vi "Write CAN Frame.vi"(7 "CAN Channel":u16=1, 8 "error in (no error)":errorcluster, 10 "CAN Frame":T1 {"type" items=["CAN Data"=0, "CAN Remote"=1, "CAN Bus Error"=2, "CAN 2.0 Data"=8, "CAN FD Data"=16, "CAN FD+BRS Data"=24, "J1939 Data"=192, "Delay"=224, "Log Trigger"=225, "Start Trigger"=226]; "payload" format="%x"; "timestamp" format="%<%.7X\n%x>T"; "identifier" format="%x"}, 11 "BLF File In":refnum<class "Read Write BLF.lvclass">) -> (0 "error out":errorcluster, 3 "BLF File Out":refnum<class "Read Write BLF.lvclass">)   [LabVIEW 2015, in "Read Write BLF.lvclass"]
doc: "This VI will write a single <B>CAN frame</B> to a BLF File.\n\n-------------\nBrian Hoover (Hooovahh)"
uses:
  Read Write BLF.lvclass
  Controls/Cluster - CAN Frame.ctl
  Controls/Enum - CAN Data Type.ctl
  Read Write BLF.lvclass/Read Write BLF.ctl
  Controls/Cluster - CAN Message.ctl
  Controls/Cluster - mHeader.ctl
  Controls/Cluster - mHeaderBase.ctl
  Controls/Enum - Read Object Types.ctl
  <vilib>/Utility/error.llb/Error Cluster From Error Code.vi
  <vilib>/Utility/libraryn.llb/Check if File or Folder Exists.vi
  SubVIs/BasicAppPath.vi
  <vilib>/ErrorRing/Error Ring.xnode
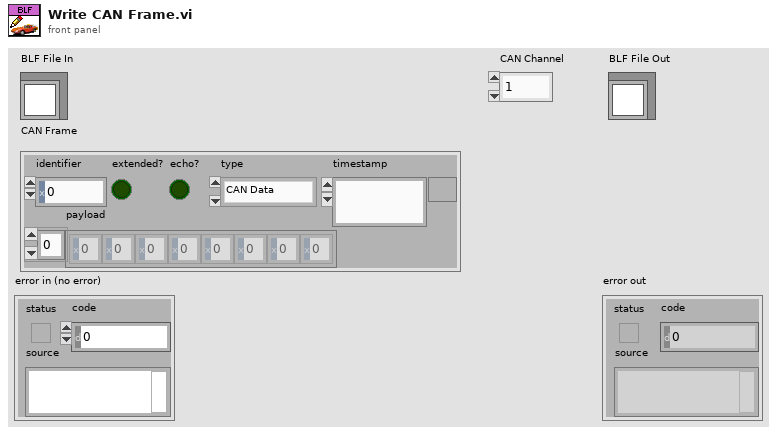
[diagram p1: front panel]
types:
  T1 = typedef "Read Write BLF.lvclass/Cluster - CAN Frame.ctl" = cluster{"timestamp":timestamp, "payload":u8[], "identifier":u32, "extended?":bool, "echo?":bool, "type":T2}
  T2 = typedef "Read Write BLF.lvclass/Enum - CAN Data Type.ctl" = u8
  T3 = typedef "Read Write BLF.lvclass/Cluster - mHeader.ctl" = cluster{"mHeaderBase":T4, "mObjectFlags":u32, "mReserved":u16, "mObjectVersion":u16, "mObjectTimeStamp":u64}
  T4 = typedef "Read Write BLF.lvclass/Cluster - mHeaderBase.ctl" = cluster{"mSignature":u32, "mHeaderSize":u16, "mHeaderVersion":u16, "mObjectSize":u32, "Object Type":T5}
  T5 = typedef "Read Write BLF.lvclass/Enum - Read Object Types.ctl" = enum32{"UNKNOWN", "CAN_MESSAGE", "CAN_ERROR", "CAN_OVERLOAD", "CAN_STATISTIC", "APP_TRIGGER", "ENV_INTEGER", "ENV_DOUBLE", "ENV_STRING", "ENV_DATA", "LOG_CONTAINER", "LIN_MESSAGE", "LIN_CRC_ERROR", "LIN_DLC_INFO", "LIN_RCV_ERROR", "LIN_SND_ERROR", "LIN_SLV_TIMEOUT", "LIN_SCHED_MODCH", "LIN_SYN_ERROR", "LIN_BAUDRATE", "LIN_SLEEP", "LIN_WAKEUP", "MOST_SPY", "MOST_CTRL", "MOST_LIGHTLOCK", "MOST_STATISTIC", "reserved_1", "reserved_2", "reserved_3", "FLEXRAY_DATA", "FLEXRAY_SYNC", "CAN_DRIVER_ERROR", "MOST_PKT", "MOST_PKT2", "MOST_HWMODE", "MOST_REG", "MOST_GENREG", "MOST_NETSTATE", "MOST_DATALOST", "MOST_TRIGGER", "FLEXRAY_CYCLE", "FLEXRAY_MESSAGE", "LIN_CHECKSUM_INFO", "LIN_SPIKE_EVENT", "CAN_DRIVER_SYNC", "FLEXRAY_STATUS", "GPS_EVENT", "FR_ERROR", "FR_STATUS", "FR_STARTCYCLE", "FR_RCVMESSAGE", "REALTIMECLOCK", "AVAILABLE2", "AVAILABLE3", "LIN_STATISTIC", "J1708_MESSAGE", "J1708_VIRTUAL_MSG", "LIN_MESSAGE2", "LIN_SND_ERROR2", "LIN_SYN_ERROR2", "LIN_CRC_ERROR2", "LIN_RCV_ERROR2", "LIN_WAKEUP2", "LIN_SPIKE_EVENT2", "LIN_LONG_DOM_SIG", "APP_TEXT", "FR_RCVMESSAGE_EX", "MOST_STATISTICEX", "MOST_TXLIGHT", "MOST_ALLOCTAB", "MOST_STRESS", "ETHERNET_FRAME", "SYS_VARIABLE", "CAN_ERROR_EXT", "CAN_DRIVER_ERROR_EXT", "LIN_LONG_DOM_SIG2", "MOST_150_MESSAGE", "MOST_150_PKT", "MOST_ETHERNET_PKT", "MOST_150_MESSAGE_FRAGMENT", "MOST_150_PKT_FRAGMENT", "MOST_ETHERNET_PKT_FRAGMENT", "MOST_SYSTEM_EVENT", "MOST_150_ALLOCTAB", "MOST_50_MESSAGE", "MOST_50_PKT", "CAN_MESSAGE2", "LIN_UNEXPECTED_WAKEUP", "LIN_SHORT_OR_SLOW_RESPONSE", "LIN_DISTURBANCE_EVENT", "SERIAL_EVENT", "OVERRUN_ERROR", "EVENT_COMMENT", "WLAN_FRAME", "WLAN_STATISTIC", "MOST_ECL", "GLOBAL_MARKER", "AFDX_FRAME", "AFDX_STATISTIC", "KLINE_STATUSEVENT", "CAN_FD_MESSAGE", "CAN_FD_MESSAGE_64", "ETHERNET_RX_ERROR", "ETHERNET_STATUS", "CAN_FD_ERROR_64", "LIN_SHORT_OR_SLOW_RESPONSE2", "AFDX_STATUS", "AFDX_BUS_STATISTIC"}
  T6 = typedef "Read Write BLF.lvclass/Cluster - CAN Message.ctl" = cluster{"mHeader":T3, "mChannel":u16, "mFlags":u8, "mDLC":u8, "mID":u32, "mData":cluster{"mData[0]":u8, "mData[1]":u8, "mData[2]":u8, "mData[3]":u8, "mData[4]":u8, "mData[5]":u8, "mData[6]":u8, "mData[7]":u8}}
  T7 = cluster{"payload[0]":u8, "payload[1]":u8, "payload[2]":u8, "payload[3]":u8, "payload[4]":u8, "payload[5]":u8, "payload[6]":u8, "payload[7]":u8}
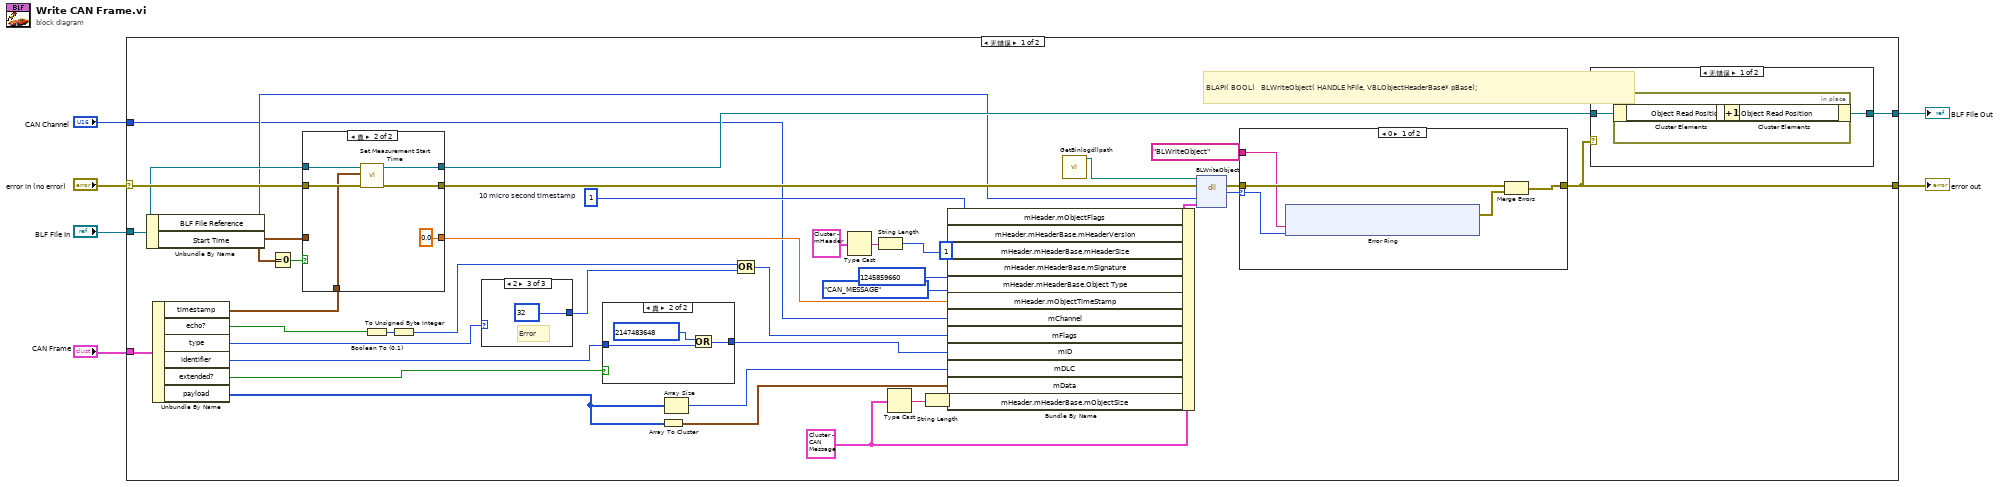
[diagram p0: block diagram]
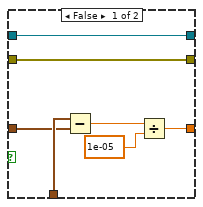
[diagram p2: hidden frame]
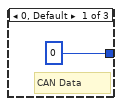
[diagram p3: hidden frame]
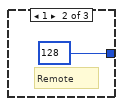
[diagram p4: hidden frame]
diagram:
  n1 = case shown="无错误" "error in (no error)" {
    selector: "error in (no error)" -> [w46 w87]
    tunnel: [w30 w87] -> w5
    tunnel: "CAN Frame" -> [w41 _]
    tunnel: "BLF File In" -> [w12 w86]
    tunnel: [w31 w86] -> w2
    tunnel: "CAN Channel" -> [w8 _]
    frame No Error {
      w15 = u8 1  # 10 micro second timestamp
      w16 = T6 {"mHeader"={"mHeaderBase"={"mSignature"=0, "mHeaderSize"=0, "mHeaderVersion"=0, "mObjectSize"=0, "Object Type"=enum."UNKNOWN"}, "mObjectFlags"=0, "mReserved"=0, "mObjectVersion"=0, "mObjectTimeStamp"=0}, "mChannel"=0, "mFlags"=0, "mDLC"=8, "mID"=0, "mData"={"mData[0]"=0, "mData[1]"=0, "mData[2]"=0, "mData[3]"=0, "mData[4]"=0, "mData[5]"=0, "mData[6]"=0, "mData[7]"=0}}
      # "BLAPI( BOOL)   BLWriteObject( HANDLE hFile, VBLObjectHeaderBase* pBase);"
      n2 = Unbundle By Name(w12) -> ("BLF File Reference"=w9:u32, "Start Time"=w14:timestamp)
      n3 = Unbundle By Name(w41) -> ("timestamp"=w34:timestamp, "echo?"=w29:bool, "type"=w27:T2, "identifier"=w40:u32, "extended?"=w39:bool, "payload"=w36:u8[])
      n4 = Equal To 0?(x=w14) -> (x = 0?=w10:bool)
      n5 = case shown="真" w10 {
        tunnel: w46 -> [w53 w58]
        tunnel: w34 -> [w52 w54]
        tunnel: [w49 0.0] -> w33
        tunnel: w14 -> [w48 _]
        tunnel: [w53 w56] -> w13
        tunnel: w12 -> [w47 w59]
        tunnel: [w47 w57] -> w11
        frame False {
          n6 = Subtract(x=w52, y=w48) -> (x-y=w51:dbl)
          n7 = Divide(x=w51, y=1e-05) -> (x/y=w49:dbl)
        }
        frame True {
          n8 = call "Set Measurement Start Time.vi"("error in (no error)"=w58, "Time Stamp (now)"=w54, "BLF File In"=w59) -> ("error out"=w56:errorcluster, "BLF File Out"=w57:refnum<class "Read Write BLF.lvclass">)  [unwired: 7 in]
        }
      }
      n9 = Boolean To (0,1)(Boolean=w29) -> (0, 1=w28:i16)
      n10 = To Unsigned Byte Integer(number=w28) -> (unsigned 8bit integer=w26:u8)
      n11 = case shown="2" w27 {
        tunnel: [u8 0 u8 128 u8 32] -> w25
        frame 0, Default {
          # "CAN Data"
        }
        frame 1 {
          # "Remote"
        }
        frame 2 {
          # "Error"
        }
      }
      n12 = case shown="真" w39 {
        tunnel: w40 -> [w68 w71]
        tunnel: [w68 w70] -> w38
        frame False {
        }
        frame True {
          n13 = Or(x=u32 2147483648, y=w71) -> (x .or. y?=w70:u32)
        }
      }
      n14 = Array To Cluster(array=w36) -> (cluster=w35:T7)
      n15 = Array Size(array=w36) -> (size(s)=w37:i32)
      n16 = Compound Arithmetic op=OR(w26, w25) -> (w32:u8)
      n17 = Type Cast(x=T3 {"mHeaderBase"={"mSignature"=0, "mHeaderSize"=0, "mHeaderVersion"=0, "mObjectSize"=0, "Object Type"=enum."UNKNOWN"}, "mObjectFlags"=0, "mReserved"=0, "mObjectVersion"=0, "mObjectTimeStamp"=0} ("mHeader")) -> (*(type *) &x=w22:string)  [unwired: 1 in]
      n18 = String Length(string=w22) -> (length=w21:i32)
      n19 = Type Cast(x=w16) -> (*(type *) &x=w18:string)  [unwired: 1 in]
      n20 = String Length(string=w18) -> (length=w17:i32)
      n21 = Bundle By Name(cluster=w16, "mHeader.mObjectFlags"=w15, "mHeader.mHeaderBase.mHeaderVersion"=u16 1, "mHeader.mHeaderBase.mHeaderSize"=w21, "mHeader.mHeaderBase.mSignature"=u32 1245859660, "mHeader.mHeaderBase.Object Type"=Enum_-_Read_Object_Types."CAN_MESSAGE", "mHeader.mObjectTimeStamp"=w33, "mChannel"=w8, "mFlags"=w32, "mID"=w38, "mDLC"=w37, "mData"=w35, "mHeader.mHeaderBase.mObjectSize"=w17) -> (w42:T6)
      n22 = call "GetBinlogdllpath.vi"() -> ("dup path"=w7:path)  [unwired: 11 in]
      n23 = dll-call lib="PTH2Vabs E自开发软件X-CAN项目 X-CAN离线分析平台 V2.2.8.0BLFbinlog.*" fn="BLWriteObject"(path in=w7, error in=w13, "hFile"=w9, "pBase"=w42) -> (error out=w44:errorcluster, "return type"=w43:i32)  [unwired: 3 in, 1 out]
      n24 = case shown="0" w43 {
        selector: w43 -> [w74 _]
        tunnel: w44 -> [w76 w85]
        tunnel: [w75 w85] -> w30
        tunnel: "BLWriteObject" -> [w73 _]
        frame 0 {
          n25 = xnode "Error Ring"("参数 0"=w73, "参数 1"=w74) -> ("错误输出"=w72:errorcluster)
          n26 = Merge Errors(w76, w72) -> (w75:errorcluster)
        }
        frame Default {
        }
      }
      n27 = case shown="无错误" w30 {
        tunnel: w11 -> [w64 w67]
        tunnel: [w63 w67] -> w31
        frame No Error {
          n28 = in-place {
            n29 = in-place-cluster #1(w64) -> ("Object Read Position"=w66:u32)
            n30 = Increment(x=w66) -> (x+1=w65:u32)
            n31 = in-place-cluster #1("Object Read Position"=w65) -> (w63:refnum<class "Read Write BLF.lvclass">)
          }
        }
        frame Error {
        }
      }
    }
    frame Error {
    }
  }
  "error out" <- w5
  "BLF File Out" <- w2
